vi "Test - Prove Pilot.vi"(8 "error in":errorcluster, 10 "Boiler Configuration":T3={"Pilot Increment (ms)"=100, "Pilot Decrement (ms)"=0}, 11 "Flame Threshold":u32=50) -> (0 "error out":errorcluster, 3 "MHL Data":T1)   [LabVIEW 2014, in "Controller.lvlib"]
uses:
  Controller.lvlib
  Boiler/Boiler Configuration.ctl
  controls/MHL UI Data.ctl
  controls/MHL Status.ctl
  Boiler/Boiler.lvlib
  support/Message Queue/Message Queue.lvlib
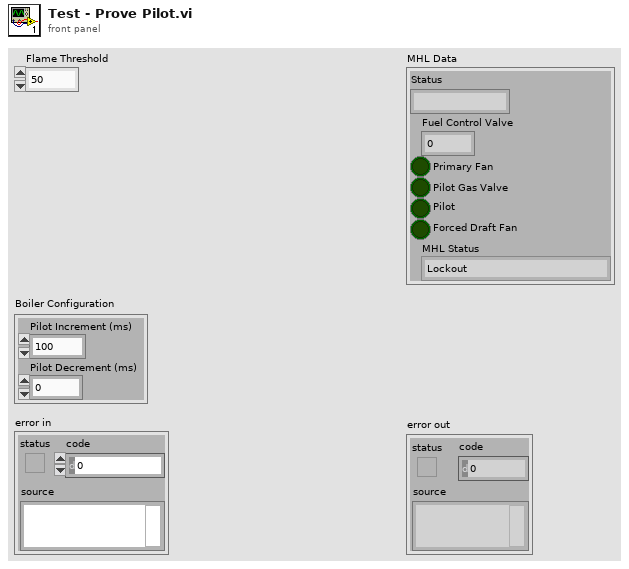
[diagram p1: front panel]
types:
  T1 = typedef "MHL UI Data.ctl" = cluster{"Status":string, "Fuel Control Valve":u32, "Primary Fan":bool, "Pilot Gas Valve":bool, "Pilot":bool, "Forced Draft Fan":bool, "MHL Status":T2}
  T2 = typedef "MHL Status.ctl" = enum16{"Lockout", "Ready", "Pre-Purge", "Pre-Purge Complete", "Pilot On", "Boiler Running", "Shutdown", "Purge"}
  T3 = typedef "Boiler.lvlib/Boiler Configuration.ctl" = cluster{"Pilot Increment (ms)":u32, "Pilot Decrement (ms)":u32}
  T4 = enum16{"open", "replace", "create", "open or create", "replace or create", "replace or create with confirmation"}
  T5 = typedef "Message Queue.lvlib/All Message Queues.ctl" = cluster{"MHL":refnum<queue>, "Boiler Controller":refnum<queue>, "Boiler":refnum<queue>}
  T6 = typedef "Notifiers.ctl" = cluster{"Handshake":refnum<notifier>, "Flame Level":refnum<notifier>, "Controller Exit":refnum<notifier>, "Boiler Exit":refnum<notifier>}
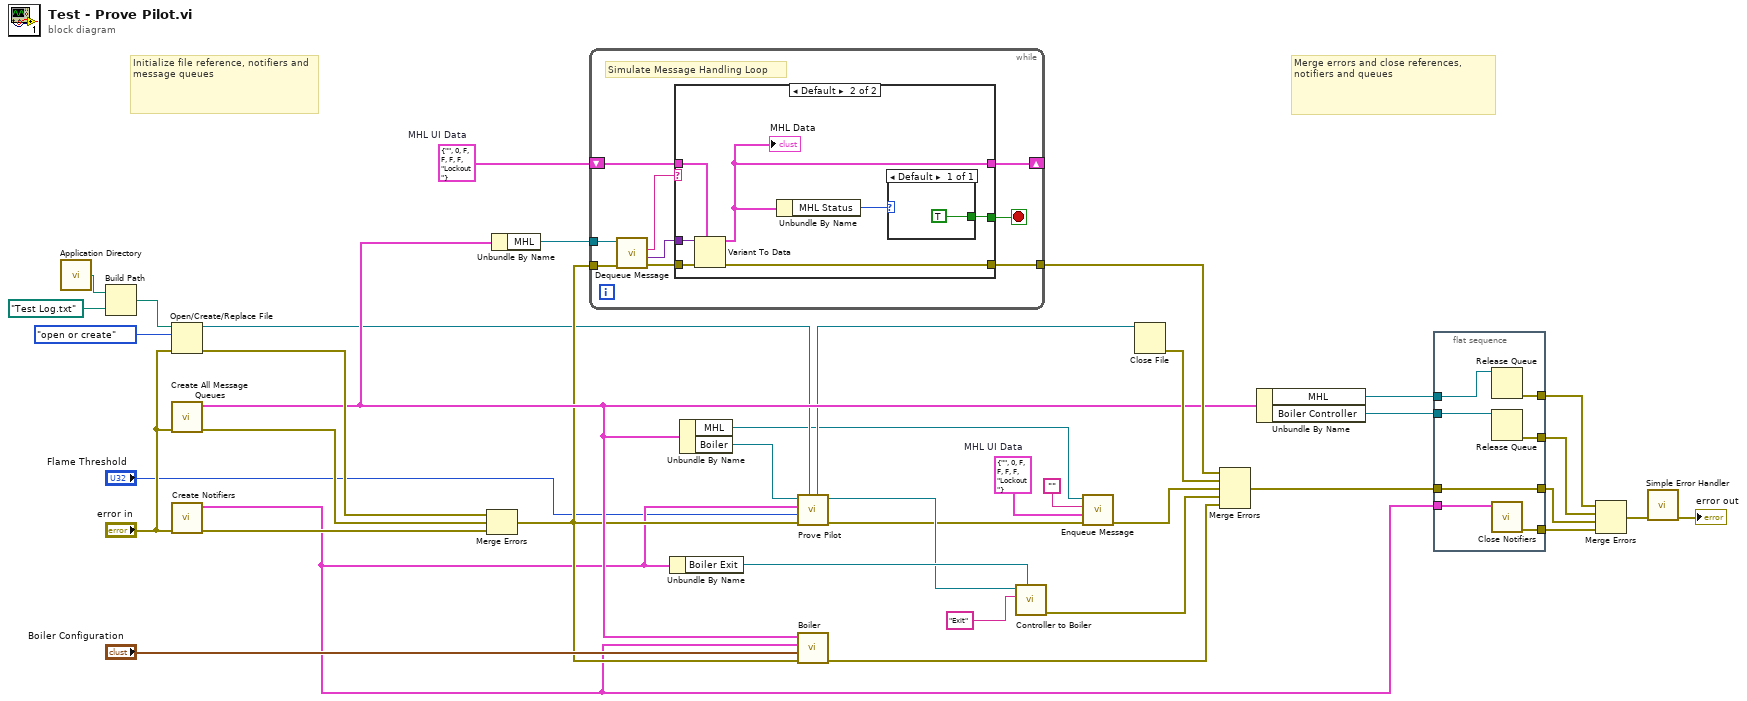
[diagram p0: block diagram]
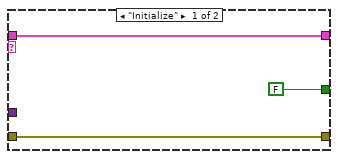
[diagram p2: hidden frame]
diagram:
  w3 = T1 {"Status"="", "Fuel Control Valve"=0, "Primary Fan"=FALSE, "Pilot Gas Valve"=FALSE, "Pilot"=FALSE, "Forced Draft Fan"=FALSE, "MHL Status"=enum."Lockout"}  # MHL UI Data
  w29 = T1 {"Status"="", "Fuel Control Valve"=0, "Primary Fan"=FALSE, "Pilot Gas Valve"=FALSE, "Pilot"=FALSE, "Forced Draft Fan"=FALSE, "MHL Status"=enum."Lockout"}  # MHL UI Data
  # "Merge errors and close references, notifiers and queues"
  # "Initialize file reference, notifiers and message queues"
  n1 = call <vilib>:"Application Directory.vi"() -> ("Application Directory"=w37:path)
  n2 = Build Path(base path=w37, name or relative path=path "Test Log.txt") -> (appended path=w35:path)
  n3 = Open/Create/Replace File(file path (use dialog)=w35, error in="error in", operation (0:open)=T4."open or create") -> (refnum out=w10:refnum<file>, error out=w33:errorcluster)  [unwired: 3 in, 1 out]
  n4 = call "Create All Message Queues.vi"("error in"="error in") -> ("error out"=w38:errorcluster, "Message Queues out"=w13:T5)  [unwired: 9 in]
  n5 = call "Create Notifiers.vi"("error in"="error in") -> ("error out"=w39:errorcluster, "Notifiers"=w11:T6)  [unwired: 9 in]
  n6 = Merge Errors(w33, w38, w39) -> (w12:errorcluster)
  n7 = Unbundle By Name(w13) -> ("MHL"=w30:refnum<queue>)
  n8 = while {
    tunnel: w30 -> [w48]
    tunnel: w12 -> [w47]
    shift-right: [w44] -> _
    shift-left: w29 -> [w45]
    tunnel: [w41] -> w25
    stop <- w40 stop-if-true
    # "Simulate Message Handling Loop"
    n9 = call "Dequeue Message.vi"("error in (no error)"=w47, "Message Queue"=w48) -> ("error out"=w42:errorcluster, "Message Data"=w46:variant, "Message"=w43:string)  [unwired: 6 in, 1 out]
    n10 = case shown="Default" w43 {
      tunnel: w42 -> [w49 w58]
      tunnel: w46 -> [_ w57]
      tunnel: w45 -> [w51 w56]
      tunnel: [w51 w55] -> w44
      tunnel: [FALSE w53] -> w40
      tunnel: [w49 w52] -> w41
      frame "Initialize" {
      }
      frame Default {
        n11 = Variant To Data(error in=w58, type=w56, Variant=w57) -> (data=w55:T1, error out=w52:errorcluster)
        "MHL Data" <- w55
        n12 = Unbundle By Name(w55) -> ("MHL Status"=w54:T2)
        n13 = case shown="Default" w54 {
          tunnel: [TRUE] -> w53
          frame Default {
          }
        }
      }
    }
  }
  n14 = Unbundle By Name(w11) -> ("Boiler Exit"=w19:refnum<notifier>)
  n15 = Unbundle By Name(w13) -> ("MHL"=w4:refnum<queue>, "Boiler"=w7:refnum<queue>)
  n16 = call "Prove Pilot.vi"("Log File Refnum in"=w10, "error in"=w12, "Flame Threshold"="Flame Threshold", "Notifiers in"=w11, "Boiler Queue in"=w7) -> ("error out"=w5:errorcluster, "Boiler Queue out"=w6:refnum<queue>, "Log File Refnum out"=w9:refnum<file>)  [unwired: 3 in, 1 out]
  n17 = call "Boiler.vi"("error in"=w12, "Boiler Configuration"="Boiler Configuration", "Notifiers"=w11, "Message Queues"=w13) -> ("error out"=w15:errorcluster)  [unwired: 7 in]
  n18 = call "Controller to Boiler.vi"("Notifier"=w19, "Message"="Exit", "Boiler Queue in"=w6) -> ("error out"=w14:errorcluster)  [unwired: 6 in, 2 out]
  n19 = call "Enqueue Message.vi"("error in (no error)"=w5, "Message Data"=w3, "Message"="", "Message Queue"=w4) -> ("error out"=w2:errorcluster)  [unwired: 6 in, 1 out]
  n20 = Close File(refnum=w9) -> (error out=w26:errorcluster)  [unwired: 1 in, 1 out]
  n21 = Merge Errors(w25, w26, w2, w14, w15) -> (w16:errorcluster)
  n22 = Unbundle By Name(w13) -> ("MHL"=w27:refnum<queue>, "Boiler Controller"=w28:refnum<queue>)
  n23 = flat-sequence {
    tunnel: w28 -> [w66]
    tunnel: w27 -> [w65]
    tunnel: [w64] -> w23
    tunnel: [w63] -> w22
    tunnel: [w62] -> w18
    tunnel: w11 -> [w61]
    tunnel: [w60] -> w17
    tunnel: w16 -> [w60]
    frame #0 {
      n24 = Release Queue(queue=w65) -> (error out=w63:errorcluster)  [unwired: 2 in, 2 out]
      n25 = Release Queue(queue=w66) -> (error out=w64:errorcluster)  [unwired: 2 in, 2 out]
      n26 = call "Close Notifiers.vi"("Notifiers"=w61) -> ("error out"=w62:errorcluster)  [unwired: 10 in]
    }
  }
  n27 = Merge Errors(w22, w23, w17, w18) -> (w21:errorcluster)
  n28 = call <vilib>:"Simple Error Handler.vi"("error in (no error)"=w21) -> ("error out"=→"error out":errorcluster)  [unwired: 4 in, 4 out]
